vi "SRV_Sensor View Tab_Make All Visible.vi"(5 "Sensor View refs":T1, 11 "error in (no error)":errorcluster, 12 "Make All Visible?":bool) -> (6 "Sensor View refs dup":T1, 15 "error out":errorcluster)   [LabVIEW 2014]
uses:
  SRV_Sensor View refs.ctl
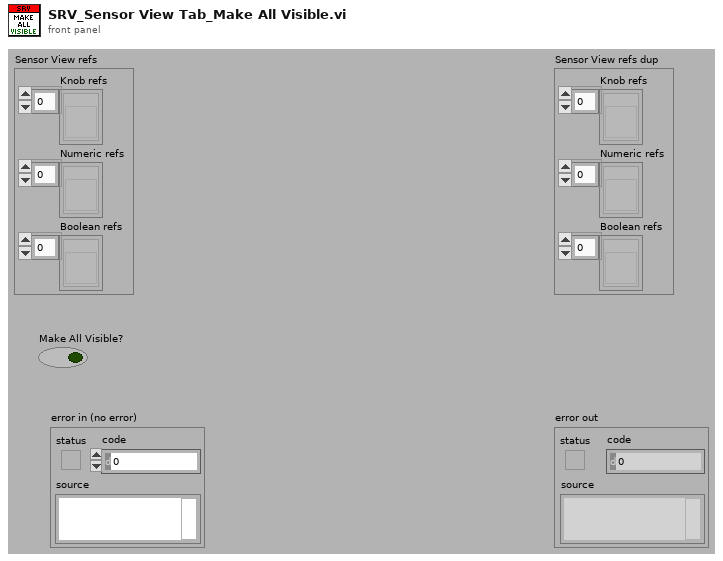
[diagram p1: front panel]
types:
  T1 = typedef "SRV_Sensor View refs.ctl" = cluster{"Knob refs":refnum<vi>[], "Numeric refs":refnum<vi>[], "Boolean refs":refnum<vi>[]}
  T2 = enum8{"Enabled", "Disabled", "Disabled and Grayed Out"}
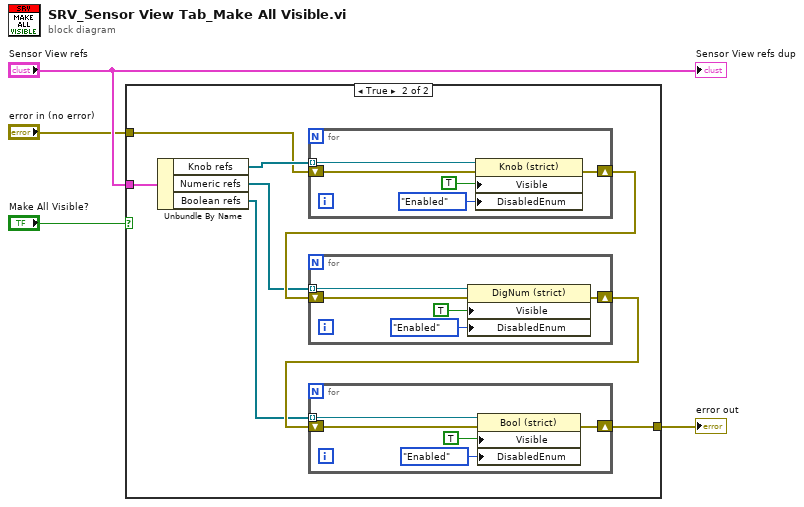
[diagram p0: block diagram]
diagram:
  n1 = case shown="True" "Make All Visible?" {
    tunnel: [w5 w8] -> w4
    tunnel: "Sensor View refs" -> [_ w7]
    tunnel: "error in (no error)" -> [w5 w6]
    frame False {
    }
    frame True {
      n2 = Unbundle By Name(w7) -> ("Knob refs"=w13:refnum<vi>[], "Numeric refs"=w10:refnum<vi>[], "Boolean refs"=w9:refnum<vi>[])
      n3 = for {
        tunnel: w13 -> [w26] mode=indexing
        shift-right: [w28] -> w12
        shift-left: w6 -> [w25]
        n4 = property class="Knob (strict)"(reference=w26, error in=w25, "Visible"=TRUE ("Caption.Visible"), "DisabledEnum"=T2."Enabled" ("Disabled")) -> (error out=w28:errorcluster)  [unwired: 1 out]
      }
      n5 = for {
        tunnel: w10 -> [w21] mode=indexing
        shift-right: [w23] -> w11
        shift-left: w12 -> [w20]
        n6 = property class="DigNum (strict)"(reference=w21, error in=w20, "Visible"=TRUE ("Caption.Visible"), "DisabledEnum"=T2."Enabled" ("Disabled")) -> (error out=w23:errorcluster)  [unwired: 1 out]
      }
      n7 = for {
        tunnel: w9 -> [w16] mode=indexing
        shift-right: [w18] -> w8
        shift-left: w11 -> [w15]
        n8 = property class="Bool (strict)"(reference=w16, error in=w15, "Visible"=TRUE ("Caption.Visible"), "DisabledEnum"=T2."Enabled" ("Disabled")) -> (error out=w18:errorcluster)  [unwired: 1 out]
      }
    }
  }
  "error out" <- w4
  "Sensor View refs dup" <- "Sensor View refs"
